vi "svx_Orbit XY Position.vi"(4 "text color":u32(colorbox), 6 "BG color":u32(colorbox)=16777216, 7 "Size":i16, 8 "text":string, 9 "angle (rad)":dbl, 10 "Plot Area:Size":T1={"Width"=100, "Height"=100}, 11 "Picture in":picture) -> (1 "text max size":i16, 2 "Plot Area:Size out":T1={"Width"=100, "Height"=100}, 3 "Picture out":picture)   [LabVIEW 2017, in "SVX Orbit.xctl"]
uses:
  <vilib>/addons/_XControls/Orbit Plot/SVX Orbit.xctl
  <vilib>/Utility/miscctls.llb/LVBoundsTypeDef.ctl
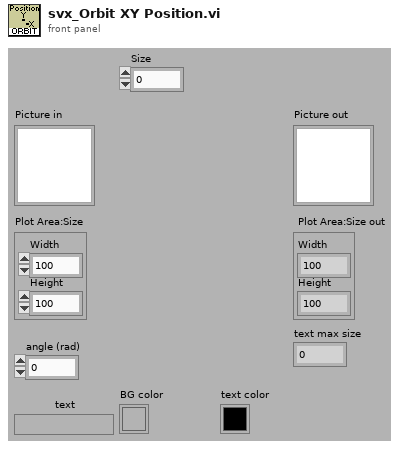
[diagram p1: front panel]
types:
  T1 = typedef "LVBoundsTypeDef.ctl" = cluster{"Width":u32, "Height":u32}
  T2 = enum16{"User-specified Font", "Application Font", "System Font", "Dialog Font"}
  T3 = cluster{"Font Name:":string, "Size":i16, "Strikeout?":bool, "Italic?":bool, "Underline?":bool, "Outline?":bool, "Shadow?":bool, "Bold?":bool}
  T4 = cluster{"left":i16, "top":i16, "right":i16, "bottom":i16}
  T5 = cluster{"horizontal":enum16{"left", "center", "right"}, "vertical":enum16{"top", "center", "bottom"}}
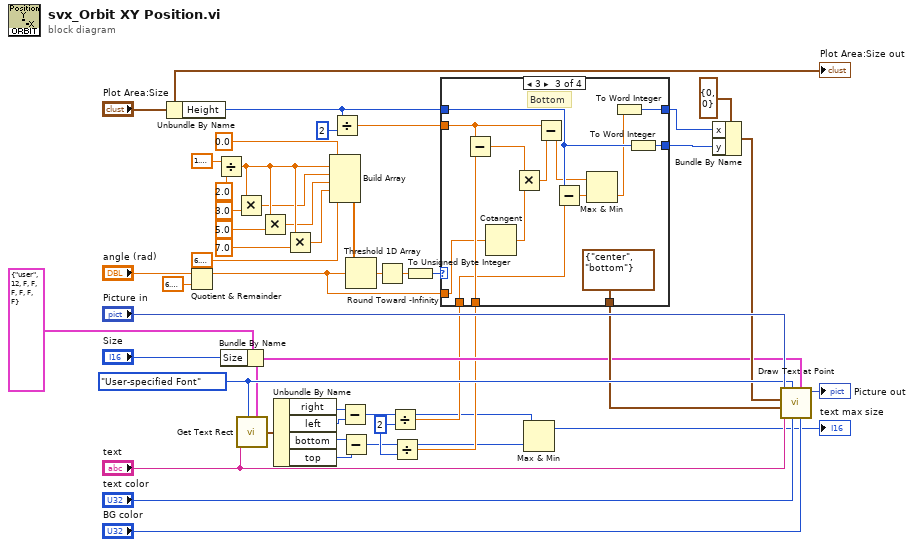
[diagram p0: block diagram]
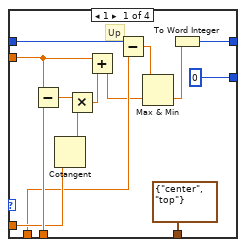
[diagram p2: hidden frame]
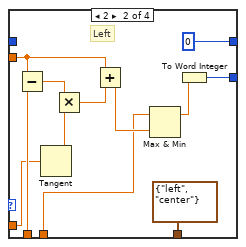
[diagram p3: hidden frame]
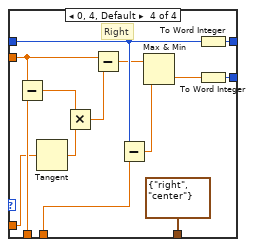
[diagram p4: hidden frame]
diagram:
  w8 = i16 2 ("y")
  w38 = T2."User-specified Font" ("desired font(Application)")
  n1 = Unbundle By Name("Plot Area:Size") -> ("Height"=w15:u32)
  n2 = Quotient & Remainder(x="angle (rad)", y=6.283185307179586) -> (x-y*floor(x/y)=w9:dbl)  [unwired: 1 out]
  n3 = Divide(x=1.5707963267948966, y=2.0) -> (x/y=w25:dbl)
  n4 = Bundle By Name(cluster=T3 {"Font Name:"="user", "Size"=12, "Strikeout?"=FALSE, "Italic?"=FALSE, "Underline?"=FALSE, "Outline?"=FALSE, "Shadow?"=FALSE, "Bold?"=FALSE} ("[user-specified font]"), "Size"="Size") -> (w7:T3)
  n5 = Multiply(x=w25, y=3.0) -> (x*y=w24:dbl)
  n6 = call <vilib>:"Get Text Rect.vi"("desired font(Application)"=w38, "text"="text", "[user-specified font]"=w7) -> ("rect"=w39:T4)  [unwired: 6 in]
  n7 = Multiply(x=w25, y=5.0) -> (x*y=w23:dbl)
  n8 = Unbundle By Name(w39) -> ("right"=w37:i16, "left"=w36:i16, "bottom"=w35:i16, "top"=w34:i16)
  n9 = Multiply(x=w25, y=7.0) -> (x*y=w22:dbl)
  n10 = Build Array(0.0 ("y"), w25, w24, w23, w22, 6.283185307179586) -> (w21:dbl[])
  n11 = Divide(x=w15, y=u32 2) -> (x/y=w10:dbl)
  n12 = Subtract(x=w37, y=w36) -> (x-y=w3:i16)
  n13 = Subtract(x=w35, y=w34) -> (x-y=w4:i16)
  n14 = Threshold 1D Array(2:w9, 3:w21) -> (0:w19:dbl)  [unwired: 1 in]
  n15 = Round Toward -Infinity(1:w19) -> (0:w18:dbl)
  n16 = Divide(x=w3, y=w8) -> (x/y=w6:dbl)
  n17 = Divide(x=w4, y=w8) -> (x/y=w5:dbl)
  n18 = To Unsigned Byte Integer(number=w18) -> (unsigned 8bit integer=w17:u8)
  n19 = case shown="3" w17 {
    tunnel: w15 -> [w51 _ w78 w92]
    tunnel: w6 -> [w50 w71 w77 w101]
    tunnel: [w53 i16 0 w82 w95] -> w14
    tunnel: [i16 0 w65 w83 w94] -> w12
    tunnel: [T5 {"horizontal"=enum."center", "vertical"=enum."top"} ("alignment(left, top)") T5 {"horizontal"=enum."left", "vertical"=enum."center"} ("alignment(left, top)") T5 {"horizontal"=enum."center", "vertical"=enum."bottom"} ("alignment(left, top)") T5 {"horizontal"=enum."right", "vertical"=enum."center"} ("alignment(left, top)")] -> w11
    tunnel: w10 -> [w57 w67 w80 w96]
    tunnel: w9 -> [w58 w70 w79 w99]
    tunnel: w5 -> [w59 w63 w86 w91]
    frame 1 {
      # "Up"
      n20 = Subtract(x=w57, y=w59) -> (x-y=w56:dbl)
      n21 = Cotangent(1:w58) -> (0:w55:dbl)
      n22 = Multiply(x=w56, y=w55) -> (x*y=w54:dbl)
      n23 = Add(x=w57, y=w54) -> (x+y=w48:dbl)
      n24 = Subtract(x=w51, y=w50) -> (x-y=w49:dbl)
      n25 = Max & Min(x=w49, y=w48) -> (min(x,y)=w52:dbl)  [unwired: 1 out]
      n26 = To Word Integer(number=w52) -> (16bit integer=w53:i16)
    }
    frame 2 {
      # "Left"
      n27 = Subtract(x=w67, y=w71) -> (x-y=w69:dbl)
      n28 = Tangent(1:w70) -> (0:w68:dbl)
      n29 = Multiply(x=w69, y=w68) -> (x*y=w66:dbl)
      n30 = Add(x=w67, y=w66) -> (x+y=w64:dbl)
      n31 = Max & Min(x=w63, y=w64) -> (max(x,y)=w62:dbl)  [unwired: 1 out]
      n32 = To Word Integer(number=w62) -> (16bit integer=w65:i16)
    }
    frame 3 {
      # "Bottom"
      n33 = Subtract(x=w80, y=w86) -> (x-y=w81:dbl)
      n34 = Cotangent(1:w79) -> (0:w85:dbl)
      n35 = Multiply(x=w81, y=w85) -> (x*y=w84:dbl)
      n36 = Subtract(x=w80, y=w84) -> (x-y=w75:dbl)
      n37 = Subtract(x=w78, y=w77) -> (x-y=w76:dbl)
      n38 = Max & Min(x=w75, y=w76) -> (min(x,y)=w74:dbl)  [unwired: 1 out]
      n39 = To Word Integer(number=w74) -> (16bit integer=w82:i16)
      n40 = To Word Integer(number=w78) -> (16bit integer=w83:i16)
    }
    frame 0, 4, Default {
      # "Right"
      n41 = Subtract(x=w96, y=w101) -> (x-y=w98:dbl)
      n42 = Tangent(1:w99) -> (0:w97:dbl)
      n43 = Multiply(x=w98, y=w97) -> (x*y=w93:dbl)
      n44 = Subtract(x=w96, y=w93) -> (x-y=w90:dbl)
      n45 = Subtract(x=w92, y=w91) -> (x-y=w89:dbl)
      n46 = Max & Min(x=w90, y=w89) -> (min(x,y)=w88:dbl)  [unwired: 1 out]
      n47 = To Word Integer(number=w92) -> (16bit integer=w95:i16)
      n48 = To Word Integer(number=w88) -> (16bit integer=w94:i16)
    }
  }
  n49 = Max & Min(x=w3, y=w4) -> (max(x,y)=→"text max size":i16)  [unwired: 1 out]
  n50 = Bundle By Name(cluster=cluster{"x":i16, "y":i16} {"x"=0, "y"=0} ("origin"), "x"=w14, "y"=w12) -> (w13:cluster{"x":i16, "y":i16})
  n51 = call <vilib>:"Draw Text at Point.vi"("BG color(transparent)"="BG color", "[user-specified font]"=w7, "text color(black)"="text color", "desired font(Application)"=w38, "text"="text", "alignment(left, top)"=w11, "origin"=w13, "picture"="Picture in") -> ("new picture"=→"Picture out":picture)  [unwired: 2 in, 1 out]
  "Plot Area:Size out" <- "Plot Area:Size"
